vi "限幅滤波.vi"(3 "限幅值":dbl=2.0 format="%#_13g", 4 "输入值":dbl, 5 "校验结果":bool) -> (0 "输出值":dbl, 1 "状态指示":bool)   [LabVIEW 2014]
doc: "限幅滤波：第k次输入值与k-1次输入值进行比较，\n当其差值绝对值在限幅值以内，则认为输入正常，\n将本次输入值送至输出值，用于与第k+1次值进行\n比较；如果差值绝对值超过限幅值，则认为输入异常\n将第k次值用第k-1次值代替送至输出值。"
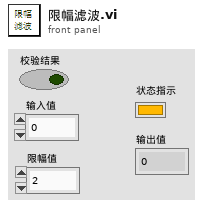
[diagram p1: front panel]
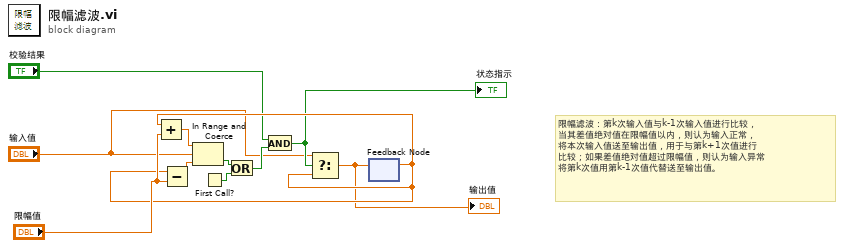
[diagram p0: block diagram]
diagram:
  # "限幅滤波：第k次输入值与k-1次输入值进行比较，\n当其差值绝对值在限幅值以内，则认为输入正常，\n将本次输入值送至输出值，用于与第k+1次值进行\n比较；如果差值绝对值超过限幅值，则认为输入异常\n将第k次值用第k-1次值代替送至输出值。"
  n1 = First Call? ("首次调用？")() -> (First Call?: T/F=w9:bool)
  n2 = feedback #1() -> (w7:dbl)  [unwired: 1 in]
  n3 = Add(x=w7, y="限幅值") -> (x+y=w5:dbl)
  n4 = Subtract(x=w7, y="限幅值") -> (x-y=w6:dbl)
  n5 = In Range and Coerce(upper limit=w5, x="输入值", lower limit=w6) -> (In Range?=w10:bool)  [unwired: 1 out]
  n6 = Or(x=w10, y=w9) -> (x .or. y?=w11:bool)
  n7 = And(x="校验结果", y=w11) -> (x .and. y?=w4:bool)
  "状态指示" <- w4
  n8 = Select(t="输入值", s=w4, f=w7) -> (s? t:f=w3:dbl)
  "输出值" <- w3
  n9 = feedback-in #1(w3) -> ()
